vi "SMR_LabVIEW_V7.61.vi"() -> ()   [LabVIEW 2025]
uses:
  <vilib>/DAQmx/write.llb/DAQmx Write (Analog DBL 1Chan 1Samp).vi
  <vilib>/DAQmx/read.llb/DAQmx Read (Analog 1D DBL NChan 1Samp).vi
  <vilib>/DAQmx/read.llb/DAQmx Read (Analog 1D DBL 1Chan NSamp).vi
  <vilib>/Analysis/baseanly.llb/Mean (DBL).vi
  <vilib>/DAQmx/create/channels.llb/DAQmx Create Channel (AI-Temperature-Thermocouple).vi
  <vilib>/DAQmx/create/channels.llb/DAQmx Create Channel (AI-Voltage-Basic).vi
  <vilib>/DAQmx/create/channels.llb/DAQmx Create Channel (AO-Voltage-Basic).vi
  <vilib>/DAQmx/miscellaneous.llb/DAQmx Fill In Error Info.vi
  <vilib>/DAQmx/configure/timing.llb/DAQmx Timing (Sample Clock).vi
  <vilib>/addons/control/pid/pid.llb/PID (DBL).vi
  <vilib>/addons/control/pid/NI_PID_pid.lvlib
  <vilib>/Analysis/NI_AALBase.lvlib
  <vilib>/ptbypt/NI_PtbyPt.lvlib
panel:
  out "Smoothed HX Flow (GPM)":dbl
  out "Voltage Across Rod (V)":dbl format="%0.2f"
  out "Current Run Folder":path
  in  "Log Root Folder":path=path "C:/Users/LocalUser/Documents/GitHub/thermal-loop/resources/v0.1.1/data/001"
  out "Raw NI9201 \nVoltage Display":T1
  in  "Loop Period (ms)":dbl=1000.0
  in  "Stop":bool
  out "Auto Steady State Threshold (deg C/min)":dbl
  out "Max dT/dt (deg C/min)":dbl
  out "Temp Change Rate (deg C/min)":dbl
  out "5-Min Baseline Complete":bool
  out "Rate Window Ready":bool
  out "Steady State":bool
  in  "Voltage Limit (V)":dbl=10.0
  in  "Temperature Limit (C)":dbl=50.0
  in  "Pressure Limit (psi)":dbl=15.0
  out "Max Voltage":bool
  out "Max Temperature":bool
  out "Max Pressure":bool
  out "Heat Exchanger Pressure History":dbl(graph)
  out "Main Loop Pressure History":T2(graph)
  out "Overall Avg Pressure (psi)":dbl
  out "Heat Exchanger Pressure P6 (psi)":dbl
  out "Main Loop Avg Pressure (psi)":dbl
  out "Pressure Display":T3
  out "Overall Pressure History":T4(graph)
  out "Max Loop Pressure (psi)":dbl
  out "Heat Exchanger Temperature History":cluster{"Waveform":dbl, "Waveform":dbl}(graph)
  out "Main Loop Temeperature History":T5(graph)
  out "Heat Exchanger Avg Temp (deg C)":dbl
  out "Temperature Display":T6
  out "Overall Temperature History":T7(graph)
  out "Overall Avg Temp (deg C)":dbl
  out "Max Loop Temp (deg C)":dbl
  out "Final P-Valve Voltage (V)":dbl
  out "PID Trim Voltage (V)":dbl
  in  "PID Temp Setpoint (deg C)":dbl
  in  "Auto PID Enable":bool
  in  "Manual P-Valve Voltage (V)":dbl min=0.0 max=10.0
  out "Main Loop Avg Temp (deg C)":dbl
  out "Flow History":dbl(graph)
  out "HX Flow (GPM)":dbl
  # "Control/Troubleshoot"
  # "Steady State"
  # "Emergency Indicators"
  # "Pressure"
  # "Temperature"
  # "Proportional Valve Control"
  # "Heat Exchanger Flow"
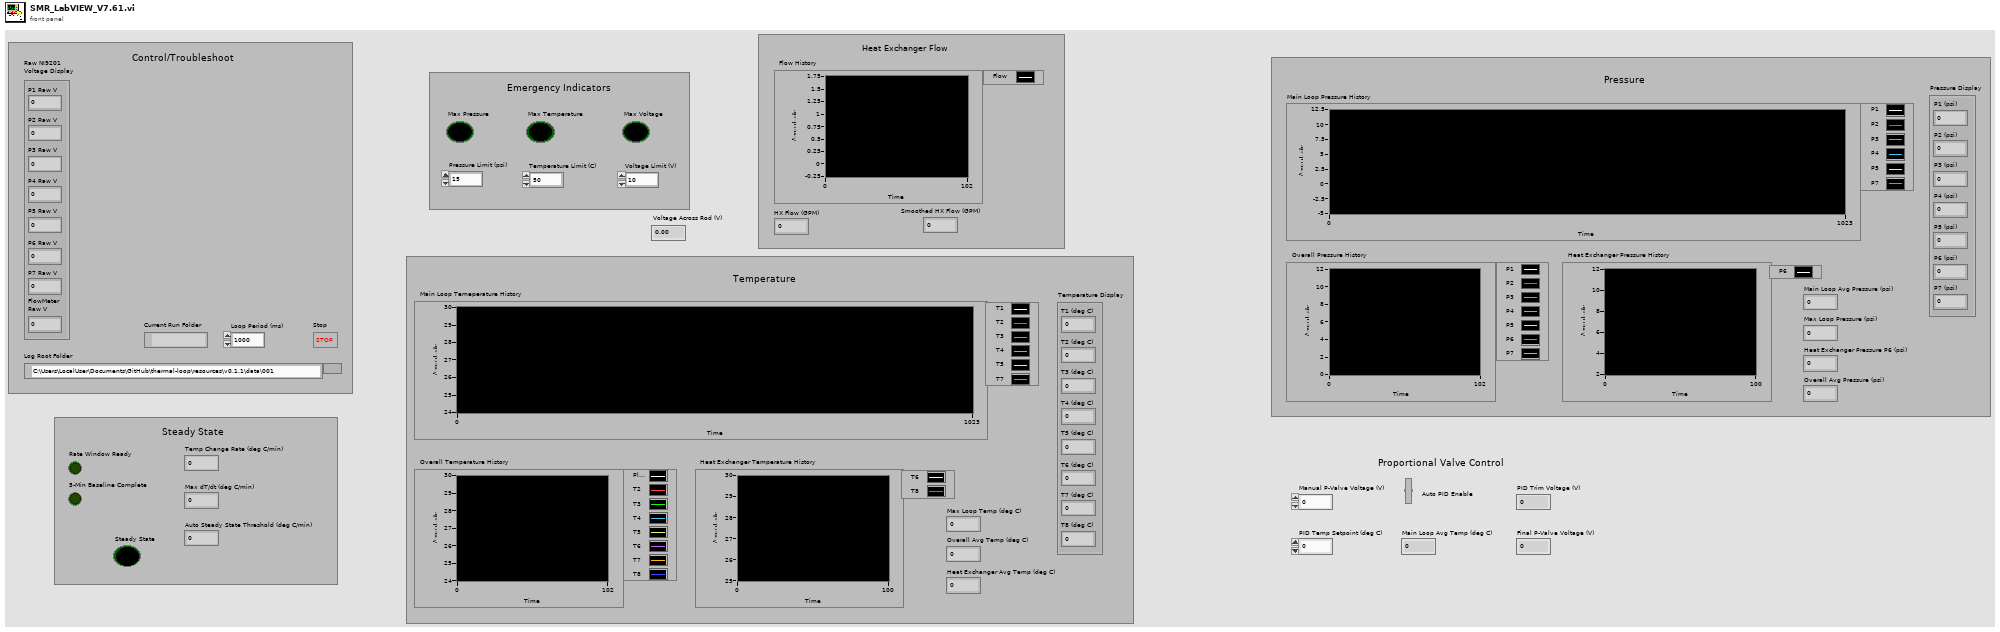
[diagram p1: front panel]
types:
  T1 = cluster{"P1 Raw V":dbl, "P2 Raw V":dbl, "P3 Raw V":dbl, "P4 Raw V":dbl, "P5 Raw V":dbl, "P6 Raw V":dbl, "P7 Raw V":dbl, "FlowMeter\nRaw V":dbl}
  T2 = cluster{"P1":dbl, "P2":dbl, "P3":dbl, "P4":dbl, "P5":dbl, "P7":dbl}
  T3 = cluster{"P1 (psi)":dbl, "P2 (psi)":dbl, "P3 (psi)":dbl, "P4 (psi)":dbl, "P5 (psi)":dbl, "P6 (psi)":dbl, "P7 (psi)":dbl}
  T4 = cluster{"P1":dbl, "P2":dbl, "P3":dbl, "P4":dbl, "P5":dbl, "P6":dbl, "P7":dbl}
  T5 = cluster{"Waveform":dbl, "Waveform":dbl, "Waveform":dbl, "Waveform":dbl, "Waveform":dbl, "Waveform":dbl}
  T6 = cluster{"T1 (deg C)":dbl, "T2 (deg C)":dbl, "T3 (deg C)":dbl, "T4 (deg C)":dbl, "T5 (deg C)":dbl, "T6 (deg C)":dbl, "T7 (deg C)":dbl, "T8 (deg C)":dbl}
  T7 = cluster{"Waveform":dbl, "Waveform":dbl, "Waveform":dbl, "Waveform":dbl, "Waveform":dbl, "Waveform":dbl, "Waveform":dbl, "Waveform":dbl}
  T8 = enum16{"open", "replace", "create", "open or create", "replace or create", "replace or create with confirmation"}
  T9 = cluster{"proportional gain (Kc)":dbl, "integral time (Ti, min)":dbl, "derivative time (Td, min)":dbl}
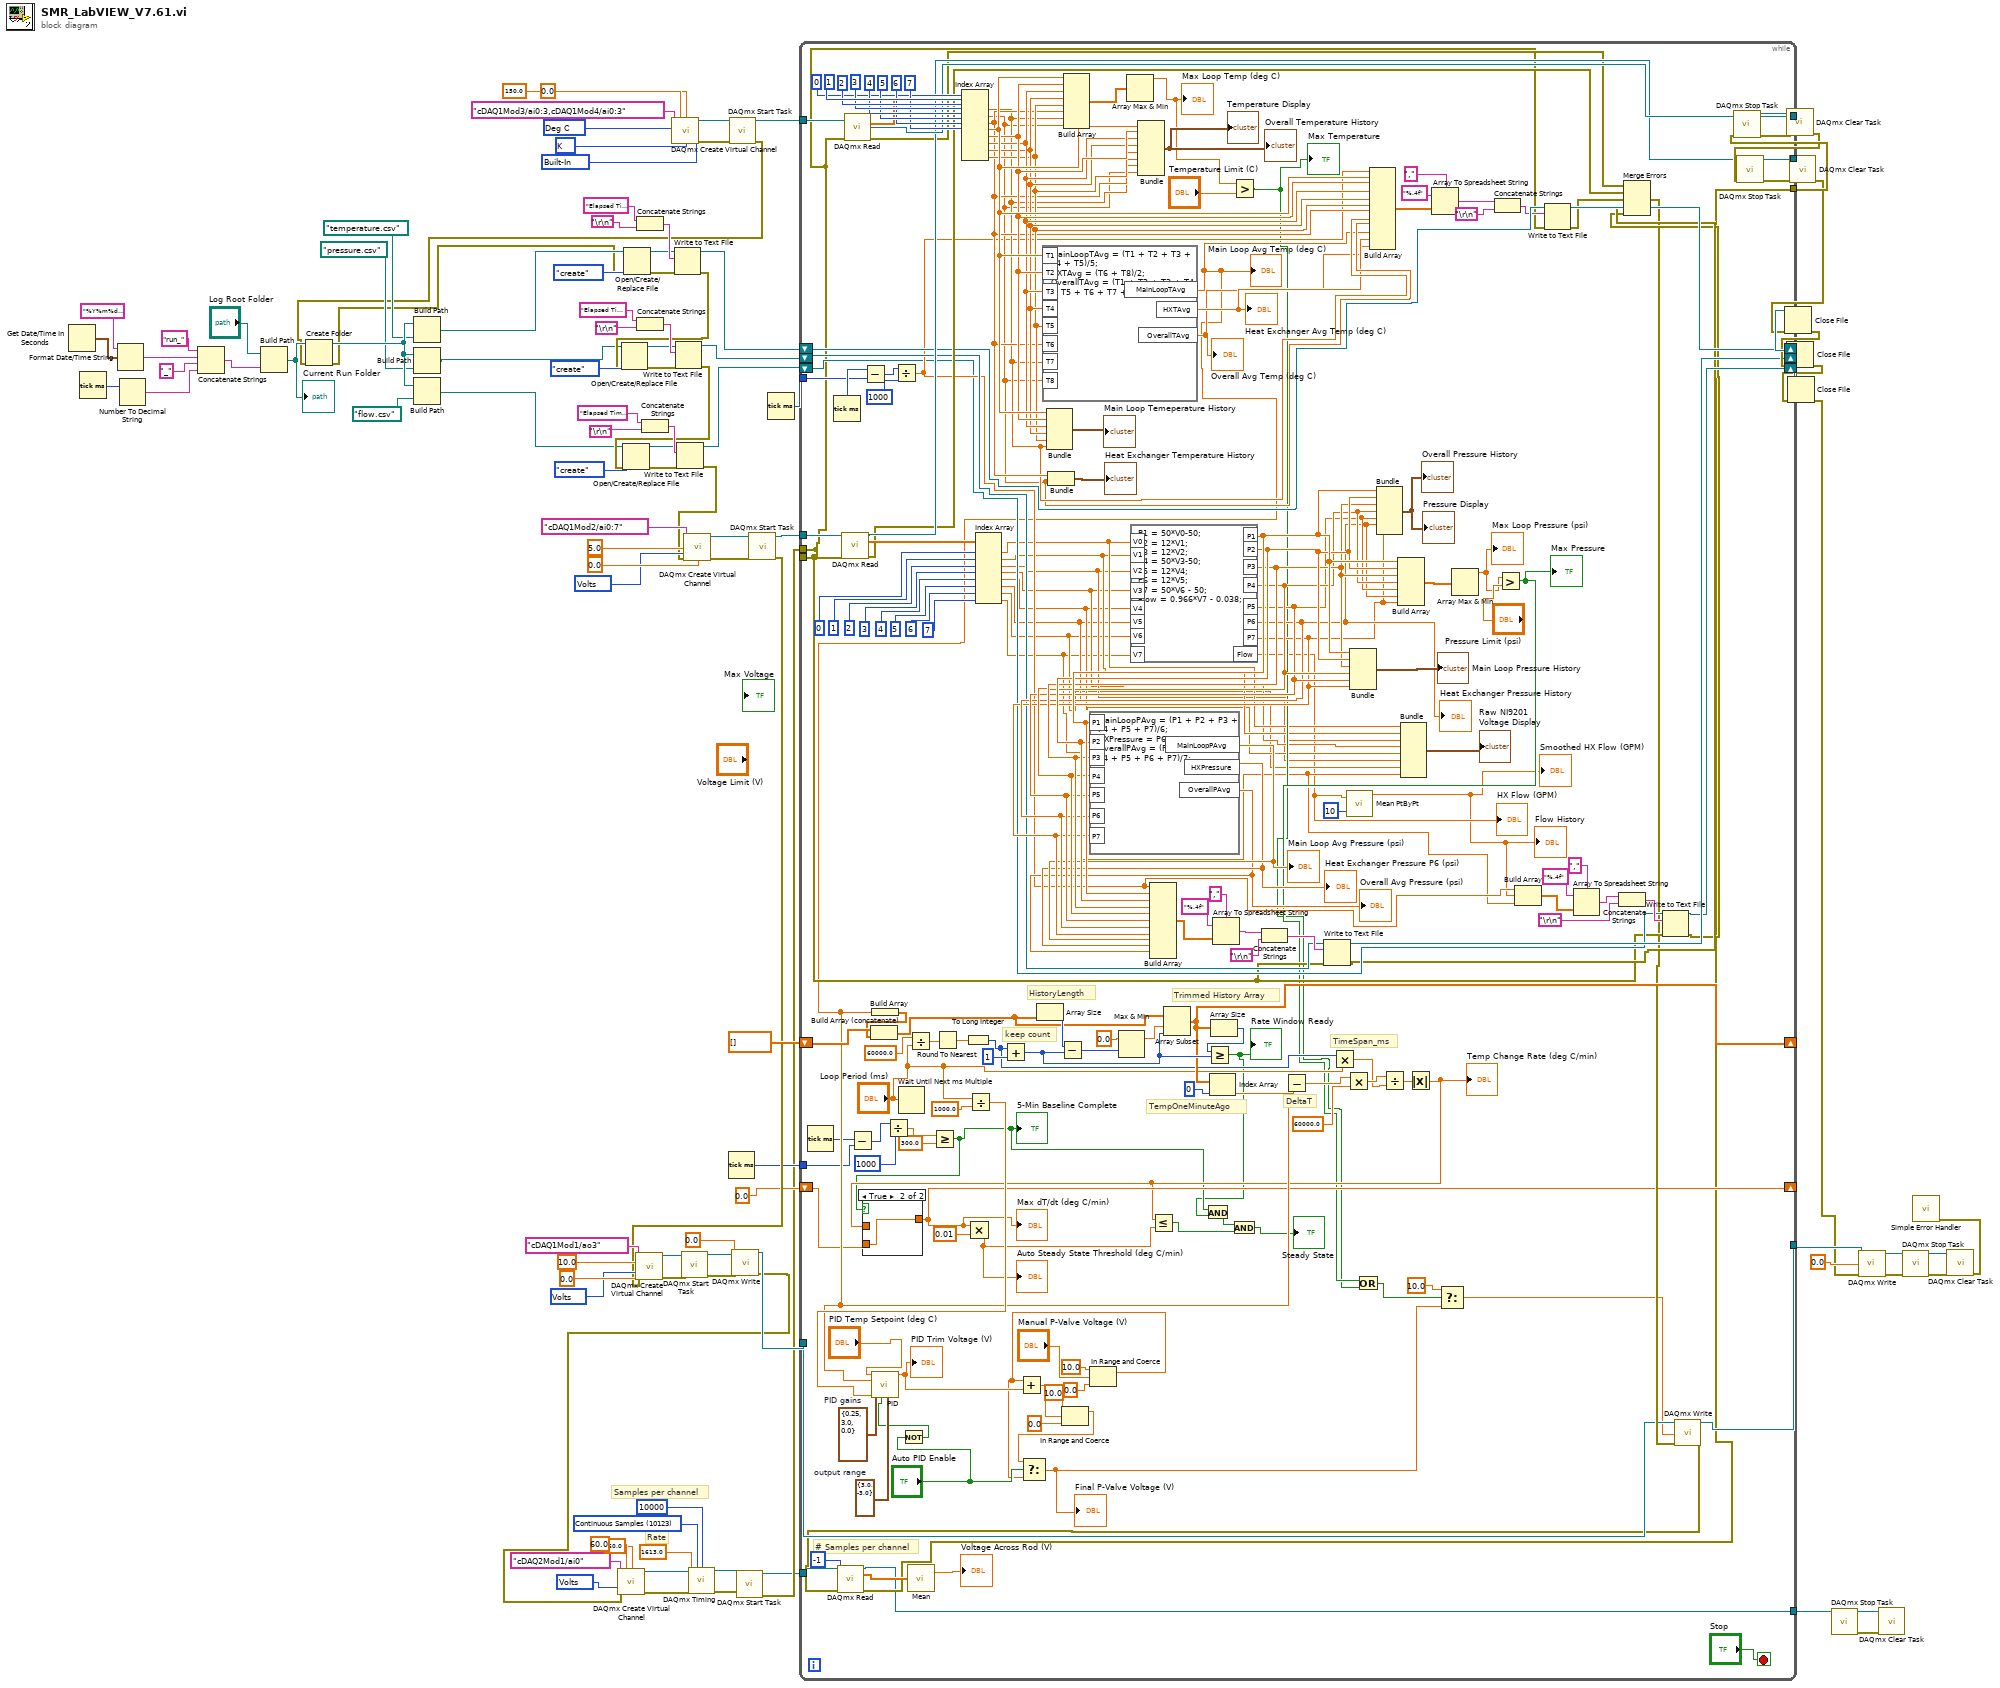
[diagram p0: block diagram]
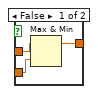
[diagram p2: hidden frame]
diagram:
  w12 = 10123 items=["Finite Samples"=10178, "Continuous Samples"=10123, "Hardware Timed Single Point"=12522] ("sample mode")
  w14 = 10348 items=["Volts"=10348, "From Custom Scale"=10065] ("units")
  w35 = 10348 items=["Volts"=10348, "From Custom Scale"=10065] ("units")
  w101 = 10200 items=["Built-In"=10200, "Constant Value"=10116, "Channel"=10113] ("cjc source")
  w102 = 10073 items=["J"=10072, "K"=10073, "N"=10077, "R"=10082, "S"=10085, "T"=10086, "B"=10047, "E"=10055] ("thermocouple type")
  w103 = 10143 items=["Deg C"=10143, "Deg F"=10144, "Kelvins"=10325, "Deg R"=10145, "From Custom Scale"=10065] ("units")
  w110 = 10348 items=["Volts"=10348, "From Custom Scale"=10065] ("units")
  # "Samples per channel"
  # "Rate"
  n1 = Get Date/Time In Seconds() -> (seconds since 1Jan1904=w58:timestamp)
  n2 = Tick Count (ms)() -> (millisecond timer value=w56:u32)
  n3 = Format Date/Time String(time format string (%c)="%Y%m%d_%H%M%S", seconds (now)=w58) -> (date/time string=w53:string)  [unwired: 1 in]
  n4 = Number To Decimal String(number=w56) -> (decimal integer string=w54:string)  [unwired: 1 in]
  n5 = Concatenate Strings("run_" ("string"), w53, "_" ("string"), w54) -> (w50:string)
  n6 = Build Path(base path="Log Root Folder", name or relative path=w50) -> (appended path=w49:path)
  "Current Run Folder" <- w49
  n7 = Concatenate Strings("Elapsed Time (s),T1 (deg C),T2 (deg C),T3 (deg C),T4 (deg C),T5 (deg C),T6 (deg C),T7 (deg C),T8 (deg C),Main Loop Avg Temp (deg C),HX Avg Temp (deg C),Overall Avg Temp (deg C)", "\r\n") -> (w84:string)
  n8 = Concatenate Strings("Elapsed Time (s),P1 (psi),P2 (psi),P3 (psi),P4 (psi),P5 (psi),P6 (psi),P7 (psi),Main Loop Avg Pressure (psi),HX Pressure (psi),Overall Avg Pressure (psi)", "\r\n") -> (w82:string)
  n9 = Concatenate Strings("Elapsed Time (s),Heat Exchanger Flow (GPM),Flow Raw Voltage (V)", "\r\n") -> (w78:string)
  n10 = call-poly <vilib>:"DAQmx Create Virtual Channel.vi"("maximum value"=150.0, "minimum value"=0.0, "physical channels"=tag "cDAQ1Mod3/ai0:3,cDAQ1Mod4/ai0:3", "cjc source"=w101, "units"=w103, "thermocouple type"=w102) -> ("task out"=w100:refnum<k21>, "error out"=w99:errorcluster)  [unwired: 8 in]
  n11 = Tick Count (ms)() -> (millisecond timer value=w19:u32)
  n12 = call <vilib>:"DAQmx Start Task.vi"("task/channels in"=w100, "error in"=w99) -> ("task out"=w98:refnum<k21>, "error out"=w41:errorcluster)  [unwired: 12 in]
  n13 = Create Folder(path (use dialog)=w49, error in=w41) -> (created path=w48:path, error out=w40:errorcluster)  [unwired: 1 in, 1 out]
  n14 = Build Path(base path=w48, name or relative path=path "temperature.csv") -> (appended path=w47:path)
  n15 = Build Path(base path=w48, name or relative path=path "pressure.csv") -> (appended path=w46:path)
  n16 = Build Path(base path=w48, name or relative path=path "flow.csv") -> (appended path=w45:path)
  n17 = Open/Create/Replace File(file path (use dialog)=w47, error in=w40, operation (0:open)=T8."create") -> (refnum out=w83:refnum<file>, error out=w67:errorcluster)  [unwired: 3 in, 1 out]
  n18 = Write to Text File(file (use dialog)=w83, text=w84, error in=w67) -> (refnum out=w74:refnum<file>, error out=w66:errorcluster)  [unwired: 1 in, 1 out]
  n19 = Open/Create/Replace File(file path (use dialog)=w46, error in=w66, operation (0:open)=T8."create") -> (refnum out=w81:refnum<file>, error out=w65:errorcluster)  [unwired: 3 in, 1 out]
  n20 = Write to Text File(file (use dialog)=w81, text=w82, error in=w65) -> (refnum out=w73:refnum<file>, error out=w64:errorcluster)  [unwired: 1 in, 1 out]
  n21 = Open/Create/Replace File(file path (use dialog)=w45, error in=w64, operation (0:open)=T8."create") -> (refnum out=w77:refnum<file>, error out=w63:errorcluster)  [unwired: 3 in, 1 out]
  n22 = Write to Text File(file (use dialog)=w77, text=w78, error in=w63) -> (refnum out=w72:refnum<file>, error out=w62:errorcluster)  [unwired: 1 in, 1 out]
  n23 = call-poly <vilib>:"DAQmx Create Virtual Channel.vi"("maximum value"=5.0, "minimum value"=0.0, "physical channels"=tag "cDAQ1Mod2/ai0:7", "units"=w110, "error in"=w62) -> ("task out"=w109:refnum<k21>, "error out"=w108:errorcluster)  [unwired: 9 in]
  n24 = call <vilib>:"DAQmx Start Task.vi"("task/channels in"=w109, "error in"=w108) -> ("task out"=w107:refnum<k21>, "error out"=w28:errorcluster)  [unwired: 12 in]
  n25 = call-poly <vilib>:"DAQmx Create Virtual Channel.vi"("maximum value"=10.0, "minimum value"=0.0, "physical channels"=tag "cDAQ1Mod1/ao3", "units"=w35, "error in"=w28) -> ("task out"=w34:refnum<k21>, "error out"=w33:errorcluster)  [unwired: 9 in]
  n26 = call <vilib>:"DAQmx Start Task.vi"("task/channels in"=w34, "error in"=w33) -> ("task out"=w32:refnum<k21>, "error out"=w31:errorcluster)  [unwired: 12 in]
  n27 = call-poly <vilib>:"DAQmx Write.vi"("task/channels in"=w32, "data"=0.0, "error in"=w31) -> ("task out"=w29:refnum<k21>, "error out"=w6:errorcluster)  [unwired: 10 in, 1 out]
  n28 = call-poly <vilib>:"DAQmx Create Virtual Channel.vi"("maximum value"=60.0, "minimum value"=-60.0, "physical channels"=tag "cDAQ2Mod1/ai0", "units"=w14, "error in"=w6) -> ("task out"=w3:refnum<k21>, "error out"=w5:errorcluster)  [unwired: 9 in]
  n29 = call-poly <vilib>:"DAQmx Timing.vi"("task/channels in"=w3, "sample mode"=w12, "samples per channel"=10000, "rate"=1613.0, "error in"=w5) -> ("task out"=w10:refnum<k21>, "error out"=w9:errorcluster)  [unwired: 9 in]
  n30 = call <vilib>:"DAQmx Start Task.vi"("task/channels in"=w10, "error in"=w9) -> ("task out"=w2:refnum<k21>, "error out"=w4:errorcluster)  [unwired: 12 in]
  n31 = Tick Count (ms)() -> (millisecond timer value=w71:u32)
  n32 = while {
    tunnel: w107 -> [w284]
    tunnel: w98 -> [w267]
    tunnel: [w257] -> w97
    tunnel: [w173] -> _
    tunnel: [w256] -> w96
    tunnel: [w127] -> w95
    shift-right: [w233] -> w70
    shift-left: w74 -> [w234]
    shift-right: [w214] -> w69
    shift-left: w73 -> [w215]
    shift-right: [w205] -> w68
    shift-left: w72 -> [w206]
    tunnel: w71 -> [w252]
    shift-right: [w184] -> _
    shift-left: dbl[] [] -> [w197]
    tunnel: w29 -> [w164]
    tunnel: w4 -> [w173]
    tunnel: [w171] -> w26
    tunnel: w19 -> [w153]
    shift-right: [w146] -> _
    shift-left: 0.0 -> [w148]
    tunnel: w2 -> [w126]
    tunnel: [w125] -> w1
    stop <- "Stop" stop-if-true
    w169 = cluster{"output high":dbl, "output low":dbl} {"output high"=3.0, "output low"=-3.0}  # output range
    w170 = T9 {"proportional gain (Kc)"=0.25, "integral time (Ti, min)"=3.0, "derivative time (Td, min)"=0.0}  # PID gains
    # "# Samples per channel"
    # "TimeSpan_ms"
    # "DeltaT"
    # "TempOneMinuteAgo"
    # "Trimmed History Array"
    # "HistoryLength"
    # "keep count"
    n33 = Tick Count (ms)() -> (millisecond timer value=w154:u32)
    n34 = Tick Count (ms)() -> (millisecond timer value=w253:u32)
    n35 = call-poly <vilib>:"DAQmx Read.vi"("task/channels in"=w284, "error in"=w173) -> ("task out"=w256:refnum<k21>, "data"=w275:dbl[], "error out"=w254:errorcluster)  [unwired: 11 in]
    n36 = call-poly <vilib>:"DAQmx Read.vi"("task/channels in"=w267, "error in"=w173) -> ("task out"=w257:refnum<k21>, "data"=w258:dbl[], "error out"=w255:errorcluster)  [unwired: 11 in]
    n37 = Subtract(x=w154, y=w153) -> (x-y=w152:u32)
    n38 = Subtract(x=w253, y=w252) -> (x-y=w251:u32)
    n39 = Divide(x=w152, y=u32 1000) -> (x/y=w150:dbl)
    n40 = Divide(x=w251, y=u32 1000) -> (x/y=w213:dbl)
    n41 = Wait Until Next ms Multiple(millisecond multiple="Loop Period (ms)") -> ()  [unwired: 1 out]
    n42 = Not(x="Auto PID Enable") -> (.not. x?=w165:bool)
    n43 = Divide(x=60000.0, y="Loop Period (ms)") -> (x/y=w194:dbl)
    n44 = Greater Or Equal?(x=w150, y=300.0) -> (x >= y?=w143:bool)
    "5-Min Baseline Complete" <- w143
    n45 = Round To Nearest(number=w194) -> (nearest integer value=w193:dbl)
    n46 = Index Array(array=w258, index #1=0 ("index"), index #2=1 ("index"), index #3=2 ("index"), index #4=3 ("index"), index #5=4 ("index"), index #6=5 ("index"), index #7=6 ("index"), index #8=7 ("index")) -> (element #1=w243:dbl, element #2=w242:dbl, element #3=w244:dbl, element #4=w249:dbl, element #5=w248:dbl, element #6=w247:dbl, element #7=w246:dbl, element #8=w245:dbl)
    n47 = To Long Integer(number=w193) -> (32bit integer=w181:i32)
    n48 = Divide(x="Loop Period (ms)", y=1000.0) -> (x/y=w166:dbl)
    n49 = Index Array(array=w275, index #1=0 ("index"), index #2=1 ("index"), index #3=2 ("index"), index #4=3 ("index"), index #5=4 ("index"), index #6=5 ("index"), index #7=6 ("index"), index #8=7 ("index")) -> (element #1=w124:dbl, element #2=w123:dbl, element #3=w122:dbl, element #4=w121:dbl, element #5=w120:dbl, element #6=w119:dbl, element #7=w118:dbl, element #8=w117:dbl)
    n50 = Add(x=w181, y=1) -> (x+y=w186:i32)
    n51 = formula code="MainLoopTAvg = (T1 + T2 + T3 + T4 + T5)/5;\nHXTAvg = (T6 + T8)/2;\nOverallTAvg = (T1 + T2 + T3 + T4 + T5 + T6 + T7 + T8)/8;"("T1"=w249, "T2"=w248, "T3"=w247, "T4"=w246, "T5"=w245, "T6"=w244, "T7"=w243, "T8"=w242) -> ("MainLoopTAvg"=w156:dbl, "HXTAvg"=w241:dbl, "OverallTAvg"=w240:dbl)
    "Overall Avg Temp (deg C)" <- w240
    "Main Loop Avg Temp (deg C)" <- w156
    "Heat Exchanger Avg Temp (deg C)" <- w241
    n52 = Build Array(w156) -> (w196:dbl[])
    n53 = Build Array (concatenate)(w197, w196) -> (w188:dbl[])
    n54 = call-poly <vilib>:"PID.vi"("reinitialize? (F)"=w165, "output range"=w169, "dt (s)"=w166, "PID gains"=w170, "process variable"=w156, "setpoint"="PID Temp Setpoint (deg C)") -> ("output"=w163:dbl)  [unwired: 4 in, 1 out]
    "PID Trim Voltage (V)" <- w163
    n55 = Array Size(array=w188) -> (size(s)=w191:i32)
    n56 = Bundle("Waveform"=w249, "Waveform"=w248, "Waveform"=w247, "Waveform"=w246, "Waveform"=w245, "Waveform"=w243) -> (→"Main Loop Temeperature History":T5)  [unwired: 1 in]
    n57 = Bundle("Waveform"=w244, "Waveform"=w242) -> (→"Heat Exchanger Temperature History":cluster{"Waveform":dbl, "Waveform":dbl})  [unwired: 1 in]
    n58 = Subtract(x=w191, y=w186) -> (x-y=w189:i32)
    n59 = Build Array(w249, w248, w247, w246, w245, w244, w243, w242) -> (w285:dbl[])
    n60 = In Range and Coerce(upper limit=10.0, x="Manual P-Valve Voltage (V)", lower limit=0.0) -> (coerced(x)=w158:dbl)  [unwired: 1 out]
    n61 = Add(x=w158, y=w163) -> (x+y=w162:dbl)
    n62 = In Range and Coerce(upper limit=10.0, x=w162, lower limit=0.0) -> (coerced(x)=w157:dbl)  [unwired: 1 out]
    n63 = Select(t=w157, s="Auto PID Enable", f=w158) -> (s? t:f=w134:dbl)
    "Final P-Valve Voltage (V)" <- w134
    n64 = Max & Min(x=0.0, y=w189) -> (max(x,y)=w187:dbl)  [unwired: 1 out]
    n65 = Array Max & Min(array=w285) -> (max value=w199:dbl)  [unwired: 3 out]
    "Max Loop Temp (deg C)" <- w199
    n66 = formula code="P1 = 50*V0-50;\nP2 = 12*V1;\nP3 = 12*V2;\nP4 = 50*V3-50;\nP5 = 12*V4;\nP6 = 12*V5; \nP7 = 50*V6 - 50;\nFlow = 0.966*V7 - 0.038;"("V0"=w124, "V1"=w123, "V2"=w122, "V3"=w121, "V4"=w120, "V5"=w119, "V6"=w118, "V7"=w117) -> ("P1"=w232:dbl, "P2"=w231:dbl, "P3"=w230:dbl, "P4"=w229:dbl, "P5"=w228:dbl, "P6"=w227:dbl, "P7"=w226:dbl, "Flow"=w116:dbl)
    "HX Flow (GPM)" <- w116
    "Heat Exchanger Pressure History" <- w227
    n67 = formula code="MainLoopPAvg = (P1 + P2 + P3 + P4 + P5 + P7)/6;\nHXPressure = P6;\nOverallPAvg = (P1 + P2 + P3 + P4 + P5 + P6 + P7)/7;"("P1"=w232, "P2"=w231, "P3"=w230, "P4"=w229, "P5"=w228, "P6"=w227, "P7"=w226) -> ("MainLoopPAvg"=w225:dbl, "HXPressure"=w224:dbl, "OverallPAvg"=w223:dbl)
    "Overall Avg Pressure (psi)" <- w223
    "Heat Exchanger Pressure P6 (psi)" <- w224
    "Main Loop Avg Pressure (psi)" <- w225
    n68 = Bundle("Waveform"=w249, "Waveform"=w248, "Waveform"=w247, "Waveform"=w246, "Waveform"=w245, "Waveform"=w244, "Waveform"=w243, "Waveform"=w242) -> (→"Overall Temperature History" →"Temperature Display":T7)  [unwired: 1 in]
    n69 = Build Array(w213, w232, w231, w230, w229, w228, w227, w226, w225, w224, w223) -> (w222:dbl[])
    n70 = Array Subset(array=w188, index=w187, length=w186) -> (w184:dbl[])
    n71 = Index Array(array=w184, index=0) -> (element=w182:dbl)
    n72 = Array Size(array=w184) -> (size(s)=w185:i32)
    n73 = Greater Or Equal?(x=w185, y=w186) -> (x >= y?=w142:bool)
    "Rate Window Ready" <- w142
    n74 = And(x=w143, y=w142) -> (x .and. y?=w141:bool)
    n75 = Array To Spreadsheet String(delimiter (Tab)=",", array=w222, 3:"%.4f" ("format string")) -> (spreadsheet string=w218:string)
    n76 = Greater?(x=w199, y="Temperature Limit (C)") -> (0:w137:bool)
    "Max Temperature" <- w137
    n77 = Concatenate Strings(w218, "\r\n") -> (w216:string)
    n78 = Subtract(x=w156, y=w182) -> (x-y=w180:dbl)
    n79 = Write to Text File(file (use dialog)=w215, text=w216, error in=w173) -> (refnum out=w214:refnum<file>, error out=w203:errorcluster)  [unwired: 1 in, 1 out]
    n80 = Multiply(x=w181, y="Loop Period (ms)") -> (x*y=w177:dbl)
    n81 = Multiply(x=w180, y=60000.0) -> (x*y=w178:dbl)
    n82 = call <vilib>:"Mean PtByPt.vi"("x"=w116, "sample length"=10) -> ("mean"=w114:dbl)  [unwired: 2 in, 1 out]
    "Flow History" <- w114
    "Smoothed HX Flow (GPM)" <- w114
    n83 = Bundle("P1"=w232, "P2"=w231, "P3"=w230, "P4"=w229, "P5"=w228, "P7"=w226) -> (→"Main Loop Pressure History":T2)  [unwired: 1 in]
    n84 = Build Array(w213, w249, w248, w247, w246, w245, w244, w243, w242, w156, w241, w240) -> (w239:dbl[])
    n85 = Bundle("P1"=w232, "P2"=w231, "P3"=w230, "P4"=w229, "P5"=w228, "P6"=w227, "P7"=w226) -> (→"Overall Pressure History" →"Pressure Display":T4)  [unwired: 1 in]
    n86 = Divide(x=w178, y=w177) -> (x/y=w176:dbl)
    n87 = Build Array(w232, w231, w230, w229, w228, w227, w226) -> (w274:dbl[])
    n88 = Bundle("Waveform"=w124, "Waveform"=w123, "Waveform"=w122, "Waveform"=w121, "Waveform"=w120, "Waveform"=w119, "Waveform"=w118, "Waveform"=w117) -> (→"Raw NI9201 \nVoltage Display":T7)  [unwired: 1 in]
    n89 = Absolute Value(x=w176) -> (abs(x)=w145:dbl)
    "Temp Change Rate (deg C/min)" <- w145
    n90 = case shown="True" w143 {
      tunnel: w148 -> [w289 w290]
      tunnel: w145 -> [w288 _]
      tunnel: [w287 w290] -> w146
      frame False {
        n91 = Max & Min(x=w288, y=w289) -> (max(x,y)=w287:dbl)  [unwired: 1 out]
      }
      frame True {
      }
    }
    "Max dT/dt (deg C/min)" <- w146
    n92 = Multiply(x=w146, y=0.01) -> (x*y=w144:dbl)
    "Auto Steady State Threshold (deg C/min)" <- w144
    n93 = Less Or Equal?(x=w145, y=w144) -> (x <= y?=w140:bool)
    n94 = And(x=w141, y=w140) -> (x .and. y?=→"Steady State":bool)
    n95 = Array To Spreadsheet String(delimiter (Tab)=",", array=w239, 3:"%.4f" ("format string")) -> (spreadsheet string=w236:string)
    n96 = Array Max & Min(array=w274) -> (max value=w200:dbl)  [unwired: 3 out]
    "Max Loop Pressure (psi)" <- w200
    n97 = Concatenate Strings(w236, "\r\n") -> (w219:string)
    n98 = Greater?(x=w200, y="Pressure Limit (psi)") -> (0:w138:bool)
    "Max Pressure" <- w138
    n99 = Or(x=w138, y=w137) -> (x .or. y?=w132:bool)
    n100 = Select(t=10.0, s=w132, f=w134) -> (s? t:f=w133:dbl)
    n101 = Build Array(w213, w114, w117) -> (w212:dbl[])
    n102 = Write to Text File(file (use dialog)=w234, text=w219, error in=w173) -> (refnum out=w233:refnum<file>, error out=w204:errorcluster)  [unwired: 1 in, 1 out]
    n103 = Array To Spreadsheet String(delimiter (Tab)=",", array=w212, 3:"%.4f" ("format string")) -> (spreadsheet string=w208:string)
    n104 = Concatenate Strings(w208, "\r\n") -> (w207:string)
    n105 = Write to Text File(file (use dialog)=w206, text=w207, error in=w173) -> (refnum out=w205:refnum<file>, error out=w202:errorcluster)  [unwired: 1 in, 1 out]
    n106 = Merge Errors(w255, w254, w204, w203, w202) -> (w172:errorcluster)
    n107 = call-poly <vilib>:"DAQmx Write.vi"("task/channels in"=w164, "data"=w133, "error in"=w172) -> ("task out"=w171:refnum<k21>, "error out"=w128:errorcluster)  [unwired: 10 in, 1 out]
    n108 = call-poly <vilib>:"DAQmx Read.vi"("task/channels in"=w126, "number of samples per channel"=-1, "error in"=w128) -> ("task out"=w125:refnum<k21>, "data"=w130:dbl[], "error out"=w127:errorcluster)  [unwired: 10 in]
    n109 = call-poly <vilib>:"Mean.vi"("X"=w130) -> ("mean"=→"Voltage Across Rod (V)":dbl)  [unwired: 1 out]
  }
  n110 = call <vilib>:"DAQmx Stop Task.vi"("task/channels in"=w97, "error in"=w95) -> ("task out"=w94:refnum<k21>, "error out"=w92:errorcluster)  [unwired: 12 in]
  n111 = call <vilib>:"DAQmx Clear Task.vi"("task in"=w94, "error in"=w92) -> ("error out"=w91:errorcluster)  [unwired: 13 in]
  n112 = call <vilib>:"DAQmx Stop Task.vi"("task/channels in"=w96, "error in"=w91) -> ("task out"=w93:refnum<k21>, "error out"=w90:errorcluster)  [unwired: 12 in]
  n113 = call <vilib>:"DAQmx Clear Task.vi"("task in"=w93, "error in"=w90) -> ("error out"=w61:errorcluster)  [unwired: 13 in]
  n114 = Close File(refnum=w70, error in=w61) -> (error out=w60:errorcluster)  [unwired: 1 out]
  n115 = Close File(refnum=w69, error in=w60) -> (error out=w59:errorcluster)  [unwired: 1 out]
  n116 = Close File(refnum=w68, error in=w59) -> (error out=w25:errorcluster)  [unwired: 1 out]
  n117 = call <vilib>:"DAQmx Stop Task.vi"("task/channels in"=w1) -> ("task out"=w8:refnum<k21>, "error out"=w7:errorcluster)  [unwired: 13 in]
  n118 = call-poly <vilib>:"DAQmx Write.vi"("task/channels in"=w26, "data"=0.0, "error in"=w25) -> ("task out"=w24:refnum<k21>, "error out"=w22:errorcluster)  [unwired: 10 in, 1 out]
  n119 = call <vilib>:"DAQmx Clear Task.vi"("task in"=w8, "error in"=w7) -> ()  [unwired: 13 in, 1 out]
  n120 = call <vilib>:"DAQmx Stop Task.vi"("task/channels in"=w24, "error in"=w22) -> ("task out"=w23:refnum<k21>, "error out"=w21:errorcluster)  [unwired: 12 in]
  n121 = call <vilib>:"DAQmx Clear Task.vi"("task in"=w23, "error in"=w21) -> ("error out"=w20:errorcluster)  [unwired: 13 in]
  n122 = call <vilib>:"Simple Error Handler.vi"("error in (no error)"=w20) -> ()  [unwired: 4 in, 5 out]
